vi "Image Name.vi"(8 "error in (no error)":errorcluster, 11 "Interface in":refnum<class "Interface.lvclass">) -> (0 "error out":errorcluster, 2 "Image Name":string, 3 "Interface out":refnum<class "Interface.lvclass">)   [LabVIEW 2018, in "Interface.lvclass"]
uses:
  Interface.lvclass
  Interface.lvclass/Interface.ctl
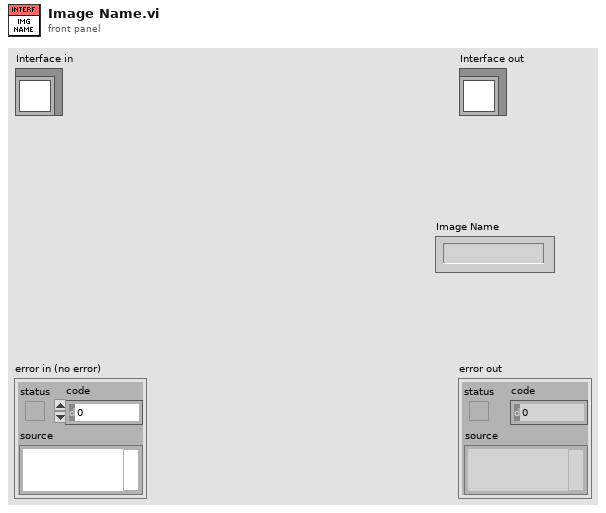
[diagram p1: front panel]
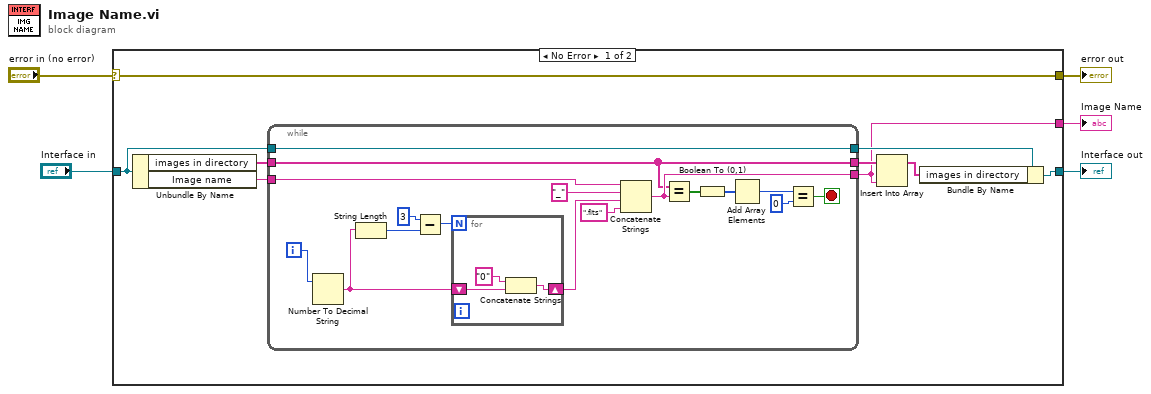
[diagram p0: block diagram]
diagram:
  n1 = case shown="No Error" "error in (no error)" {
    selector: "error in (no error)" -> [w14 w36]
    tunnel: [w14 w36] -> w4
    tunnel: [w9 w35] -> w2
    tunnel: "Interface in" -> [w12 w35]
    tunnel: [w7 _] -> w1
    frame No Error {
      n2 = Unbundle By Name(w12) -> ("images in directory"=w13:string[], "Image name"=w11:string)
      n3 = while {
        tunnel: w13 -> [w15]
        tunnel: w11 -> [w21]
        tunnel: w12 -> [w18]
        tunnel: [w18] -> w10
        tunnel: [w17] -> w7
        tunnel: [w15] -> w8
        i -> [w16]
        stop <- w20 stop-if-true
        n4 = Number To Decimal String(number=w16) -> (decimal integer string=w22:string)  [unwired: 1 in]
        n5 = String Length(string=w22) -> (length=w25:i32)
        n6 = Subtract(x=3, y=w25) -> (x-y=w26:i32)
        n7 = for {
          N: w26 -> [_]
          shift-right: [w34] -> w23
          shift-left: w22 -> [w32]
          n8 = Concatenate Strings("0" ("string"), w32) -> (w34:string)
        }
        n9 = Concatenate Strings(w21, "_" ("string"), w23, ".fits" ("string")) -> (w17:string)
        n10 = Equal?(x=w15, y=w17) -> (x = y?=w31:bool[])
        n11 = Boolean To (0,1)(Boolean=w31) -> (0, 1=w30:i16[])
        n12 = Add Array Elements(numeric array=w30) -> (sum=w29:i16)
        n13 = Equal?(x=w29, y=0) -> (x = y?=w20:bool)
      }
      n14 = Insert Into Array(array=w8, new element=w7) -> (w6:string[])  [unwired: 1 in]
      n15 = Bundle By Name(cluster=w10, "images in directory"=w6) -> (w9:refnum<class "Interface.lvclass">)
    }
    frame Error {
    }
  }
  "error out" <- w4
  "Interface out" <- w2
  "Image Name" <- w1
